vi "Position Voltage to Percent.vi"(10 "Position Sensor Output (V)":dbl) -> (2 "Cylinder Position (%)":dbl)   [LabVIEW 2015, in "cRIO-Carbondioxide.lvlib" / "CO2-Actor.lvlib" / "Cylinder.lvclass"]
uses:
  Cylinder.lvclass
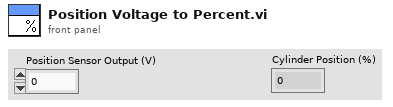
[diagram p1: front panel]
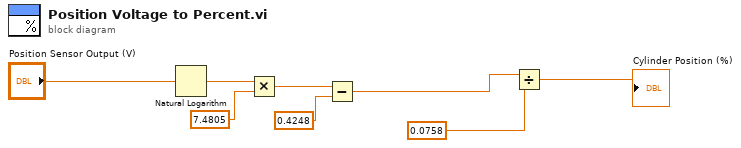
[diagram p0: block diagram]
diagram:
  n1 = Natural Logarithm(1:"Position Sensor Output (V)") -> (0:w7:dbl)
  n2 = Multiply(x=w7, y=7.4805) -> (x*y=w5:dbl)
  n3 = Subtract(x=w5, y=0.4248) -> (x-y=w1:dbl)
  n4 = Divide(x=w1, y=0.0758) -> (x/y=→"Cylinder Position (%)":dbl)
